vi "practica6.vi"() -> ()   [LabVIEW 2016]
uses:
  <vilib>/addons/Fuzzy Logic/FL Fuzzy Controller (SISO).vi
  <vilib>/addons/Fuzzy Logic/NI_Fuzzy_Logic_API.lvlib
panel:
  out "Waveform Chart":dbl[](graph)
  in  "file path 3":path
  in  "SP":dbl
  in  "stop":bool
  out "Posicion":dbl(knob)
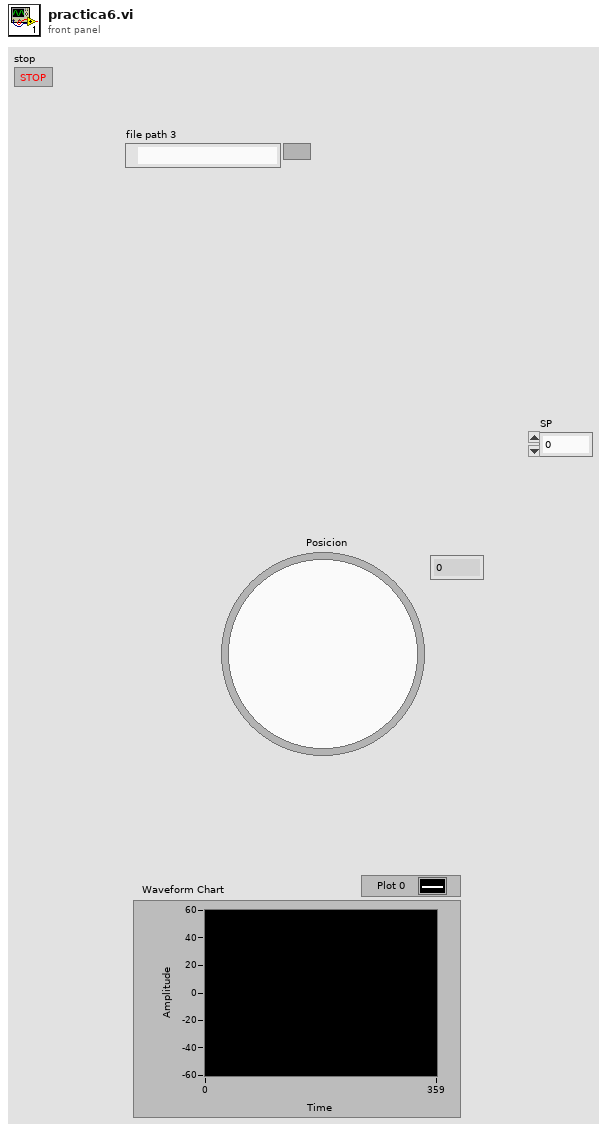
[diagram p1: front panel]
types:
  T1 = typedef "NI_Fuzzy_Logic_API.lvlib/FL System.ctl" = cluster{"input variables":T2[], "output variables":T2[], "rules":T5[], "defuzzification method":T11, "description":string, "user MF interpolating polynomials":T12[]}
  T2 = typedef "NI_Fuzzy_Logic_API.lvlib/FL Variable.ctl" = cluster{"name":string, "range":dbl[], "MFs":T3[]}
  T3 = typedef "NI_Fuzzy_Logic_API.lvlib/FL Membership Function.ctl" = cluster{"name":string, "shape":T4, "points":dbl[], "color":u32, "user-defined shape index":i32}
  T4 = typedef "NI_Fuzzy_Logic_API.lvlib/FL Membership Function Shape.ctl" = u16
  T5 = typedef "NI_Fuzzy_Logic_API.lvlib/FL Rule.ctl" = cluster{"antecedents":T6[], "antecedent connective":T8, "consequents":T9[], "consequent implication":T10, "degree of support":dbl}
  T6 = typedef "NI_Fuzzy_Logic_API.lvlib/FL Antecedent.ctl" = cluster{"Var Index":i32, "MF Index":i32, "Cond":T7}
  T7 = typedef "NI_Fuzzy_Logic_API.lvlib/FL Modifier.ctl" = u16
  T8 = typedef "NI_Fuzzy_Logic_API.lvlib/FL Antecedent Connective.ctl" = u16
  T9 = typedef "NI_Fuzzy_Logic_API.lvlib/FL Consequent.ctl" = cluster{"Var Index":i32, "MF Index":i32, "Cond":T7}
  T10 = typedef "NI_Fuzzy_Logic_API.lvlib/FL Consequent Implication.ctl" = u16
  T11 = typedef "NI_Fuzzy_Logic_API.lvlib/FL Defuzzification.ctl" = u16
  T12 = typedef "NI_Fuzzy_Logic_API.lvlib/FL Interpolating polynomials.ctl" = cluster{"X":dbl[], "Y":dbl[], "Y(x) coeff":dbl[][], "X(y) coeff":dbl[][], "Area(y) coeff":dbl[][], "coa_x(y) coeff":dbl[][]}
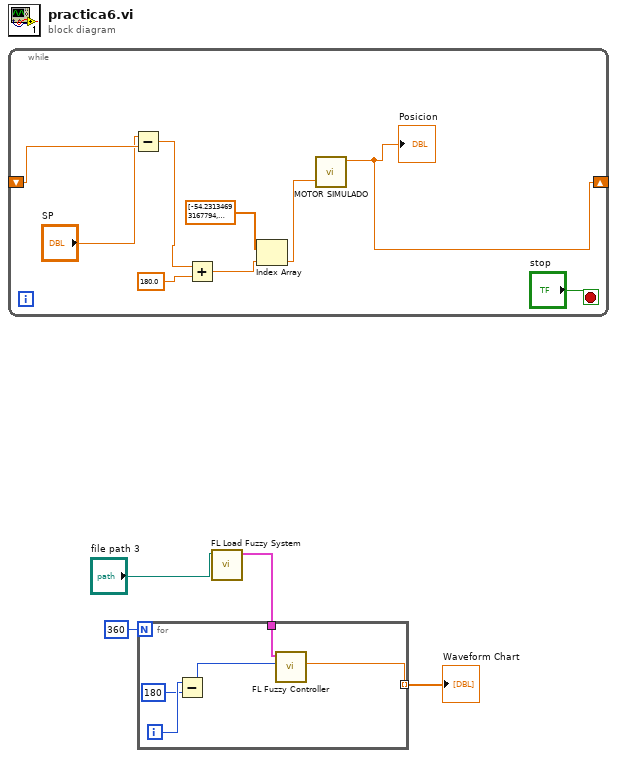
[diagram p0: block diagram]
diagram:
  n1 = while {
    shift-right: [w8] -> _
    shift-left: _ -> [w12]
    stop <- "stop" stop-if-true
    n2 = Subtract(x="SP", y=w12) -> (x-y=w7:dbl)
    n3 = Add(x=w7, y=180.0) -> (x+y=w5:dbl)
    n4 = Index Array(array=dbl[] [-54.23134693167794, -54.01981035411372, -53.8081880963361, -53.59621424441843, -53.38388792141218, -53.177457318119984, -52.97592103371202, -52.773914016032585, -52.57143461389831, -52.36848116839441, -52.16505201282931, -51.96114547268899, -51.75675986559111, -51.55189350123869, -51.34654468137356, -51.14071169972934, -50.934392841984334, -50.72758638571379, -50.52027507500864, -50.31276304218154, -50.10718558315843, -49.90111981832249, -49.694564005804054, -49.48751639543894, -49.27997522871887, -49.07193873874185, -48.87329301273477, -48.68213175723674, -48.49024973539747, -48.297642863083745, -48.10430702524765, -47.91023807563354, -47.71543183648154, -47.519884098227806, -47.32359061920141, -47.12654712531744, -46.928749309766914, -46.73008739550378, -46.539813180000515, -46.35105156771661, -46.16156129375902, -45.97133813077511, -45.78037781864868, -45.588676064181975, -45.39622854077401, -45.20303088809501, -45.00907871175708, -44.817990162314715, -44.62893603352512, -44.439003375425415, -44.24818605000184, -44.056477861928016, -43.86387255789436, -43.6703638259281, -43.47594529470389, -43.280665365876814, -43.08833479260204, -42.90001437613665, -42.710799849306646, -42.52068482935502, -42.32966287262731, -42.13772747384366, -41.94487206536029, -41.751090016420385, -41.55637463239418, -41.36071915400797, -41.16411675656193, -40.96656054913671, -40.77234309378765, -40.58026351841818, -40.386954041489986, -40.192402812319024, -39.99659782748144, -39.7995269283448, -39.60353783629167, -39.428780650149214, -39.25288175799243, -39.07582993483651, -38.89761380806438, -38.71822185499139, -38.537642400382, -38.355863613916775, -38.17287350760879, -37.98865993316829, -37.803210579314154, -37.61651296903124, -37.42855445677206, -37.239322225601605, -37.04880328428386, -36.857483194826685, -36.66510220265743, -36.66544038008633, -36.667030905439916, -36.66862399912493, -36.670219667367306, -36.6718179164131, -36.673418752528605, -36.67502218200038, -36.67662821113542, -36.67651652445535, -36.67471331251328, -36.67290127252568, -36.67819740437808, -36.686355792766605, -36.69458154336443, -36.70287549392491, -36.71123849615091, -36.71967141598639, -36.72652076403659, -36.72992436844148, -36.73336262097795, -36.73683605342107, -36.74228439478784, -36.75464995365923, -36.76716571287022, -36.77983442579346, -36.79265891351268, -36.80317431128173, -36.79826822042695, -36.79328280744587, -36.788216132929165, -36.78306619372368, -36.777830920292104, -36.79183821131308, -36.81351029943298, -36.835634809638854, -36.8582260583709, -36.86821342488431, -36.87779779963559, -36.8876106235479, -36.89766016296629, -36.90795508792422, -36.918504497090986, -36.933777473607634, -36.96456915750231, -36.99621922196928, -36.99843318212755, -36.99151500418098, -36.9843631373814, -36.97696553766131, -36.96930931883519, -36.96138067768926, -36.95316481093005, -36.944645822940466, -36.97758338551072, -37.010691954127665, -37.03330859584593, -37.057020959818026, -37.081910650502316, -37.10806758202264, -37.135591063499504, -37.16459105905095, -37.195189656163194, -37.22752278377186, -37.23821485900851, -37.23197685137446, -37.22528242444201, -37.21807958347444, -37.210308124433425, -37.20189794722042, -37.1927669352027, -37.18281826509094, -37.17193696026265, -37.14446866765724, -37.05582644657557, -37.07722896486997, -37.14592767969904, -37.224519427682125, -37.315307002471855, -37.4213680076816, -37.546910656154346, -37.697845460258286, -37.8715064719971, -37.74598245862665, -37.579978834666875, -37.414965986394556, -19.887955182072822, -10.987052885670394, -6.658196352470947, -3.094922929970275, -0.2111189303307497, 2.6071440693169694, 5.793165515233333, 9.658108404652184, 18.52741096438576, 36.054421768707485, 36.373241394650506, 36.69700493163866, 36.94386341794336, 36.997323472784075, 37.03609409256153, 37.06827786876256, 37.0954219604339, 37.11862416751464, 37.138685027665645, 37.15620205278195, 37.19143256564115, 37.277103729986315, 37.249160960438445, 37.19551803592017, 37.146485179606834, 37.101492592455436, 37.06006066177485, 37.02178279730667, 36.98631204345851, 36.95335053273681, 36.92264110094665, 36.933222785946285, 36.94653071634163, 36.95912316100076, 36.97105631033182, 36.982380620985154, 36.993141529012526, 37.003380059167284, 37.01313334757373, 37.022435091802876, 37.00827827788373, 36.9700279820564, 36.9533907383312, 36.93734732634957, 36.92186651018235, 36.90691920685785, 36.892478304011426, 36.87851849576002, 36.86501613471107, 36.847444968185776, 36.815515713078916, 36.78451940593268, 36.78357336596073, 36.79128319559412, 36.79880700975231, 36.80615146019965, 36.8133228852873, 36.82032732819723, 36.82592040244958, 36.80566619834592, 36.78579319885601, 36.76629074232663, 36.75076881620219, 36.74502636911545, 36.73937785791237, 36.733820996364514, 36.72835357183657, 36.72297344234883, 36.7099171568848, 36.69581288525711, 36.68190459035832, 36.6681882157694, 36.65465981625318, 36.654724025706216, 36.65858982994269, 36.66241651811968, 36.666204680941206, 36.66293755210737, 36.656377254291456, 36.649860525077706, 36.643386931877394, 36.63695604780975, 36.630567451608066, 36.62561396456922, 36.62421319294529, 36.62281927491983, 36.62056461754231, 36.6174338652963, 36.61431327111756, 36.61120278564776, 36.608102359847784, 36.60501194499521, 36.60193149268176, 36.598860954810746, 36.59820873343402, 36.797811257156134, 36.996603196737226, 37.19509122999284, 37.39231983553765, 37.58830096226755, 37.78304640840053, 37.976567823844185, 38.168876712519, 38.35998443463776, 38.549902208942754, 38.73864111490095, 38.9262120948588, 39.11262595615682, 39.297893373205355, 39.48202488952213, 39.66503091973236, 39.85809107546547, 40.051174121590016, 40.24308809516812, 40.433843581842964, 40.62345103984209, 40.81192080188859, 41.00095042020753, 41.191144666471985, 41.38034835906712, 41.56856921627151, 41.75581487638487, 41.94209289876135, 42.127410764826855, 42.31177587908061, 42.4951955700814, 42.677677091418595, 42.85922762266837, 43.039854270335375, 43.22937901753352, 43.42564097800257, 43.62100826286902, 43.815392019447756, 44.00879965608596, 44.20123850691355, 44.392715832770016, 44.58323882211792, 44.772814591942236, 44.96723858001855, 45.16816123855396, 45.36837444012785, 45.56788193575161, 45.766687450040216, 45.96479468144407, 46.162207302478215, 46.35892895994948, 46.554963275180825, 46.75143055150822, 46.95176680165868, 47.1513597904827, 47.35026046470112, 47.548472420154425, 47.745999227823965, 47.94284443404655, 48.13901156072651, 48.33450410554597, 48.52932554217251, 48.72347932046501, 48.91696886667733, 49.11391296249167, 49.31526829989899, 49.51607489715949, 49.71633499438764, 49.91605081952138, 50.11522458840485, 50.313858504870254, 50.516802240920505, 50.71977834622469, 50.92217566700329, 51.1240276933902, 51.325336626101034, 51.52610465402502, 51.72633395430432, 51.92602669241282, 52.12518502223402, 52.323811086138704, 52.52190701506152, 52.719474928577434, 52.91651693497705, 53.11303513134186, 53.3197176666835, 53.53855966957692, 53.757111473867084, 53.97537365640457] ("Waveform Chart 2"), index=w5) -> (element=w9:dbl)
    n5 = call "MOTOR SIMULADO.vi"("Voltaje"=w9) -> ("Posicion"=w8:dbl)  [unwired: 10 in]
    "Posicion" <- w8
  }
  n6 = call <vilib>:"FL Load Fuzzy System.vi"("file path"="file path 3") -> ("fuzzy system out"=w1:T1)  [unwired: 9 in, 1 out]
  n7 = for {
    N: 360 -> [_]
    tunnel: [w17] -> w2 mode=indexing
    tunnel: w1 -> [w18]
    i -> [w16]
    n8 = Subtract(x=w16, y=180) -> (x-y=w14:i32)
    n9 = call-poly <vilib>:"FL Fuzzy Controller.vi"("input value"=w14, "fuzzy system in"=w18) -> ("output value"=w17:dbl)  [unwired: 5 in, 4 out]
  }
  "Waveform Chart" <- w2
